vi "Read Data from converted files.vi"(10 "Open Dialog":bool=TRUE, 11 "File Control":path) -> (1 "data":dbl[][](array[numeric]), 3 "dates":string[](array[string]), 5 "File path":path)   [LabVIEW 2018]
uses:
  <vilib>/Utility/file.llb/Read From Spreadsheet File (string).vi
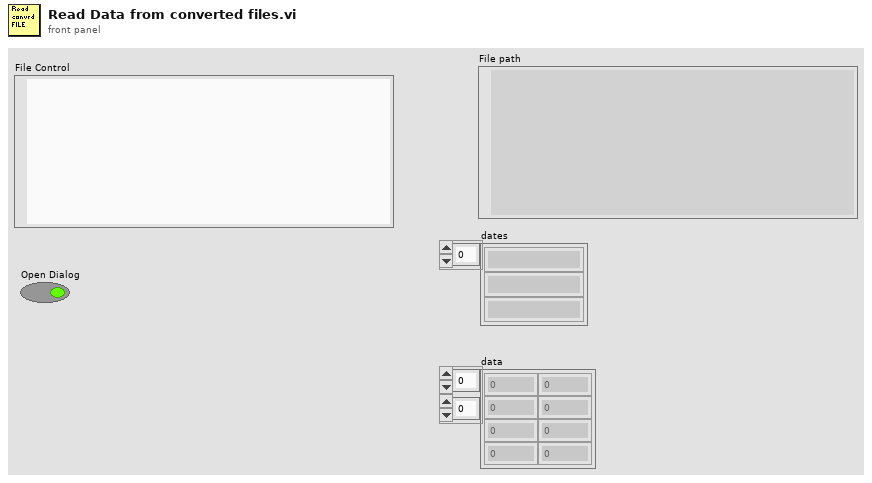
[diagram p1: front panel]
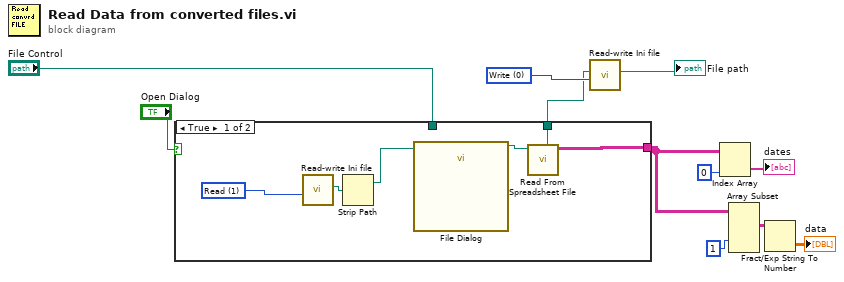
[diagram p0: block diagram]
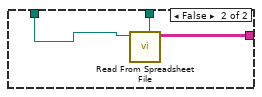
[diagram p2: hidden frame]
diagram:
  w3 = u16 0 items=["Write", "Read"] ("OPERATION")
  n1 = case shown="True" "Open Dialog" {
    tunnel: [w16 w20] -> w8
    tunnel: "File Control" -> [_ w19]
    tunnel: [w15 w18] -> w2
    frame True {
      w14 = u16 1 items=["Write", "Read"] ("OPERATION")
      n2 = call "Read-write Ini file.vi"("OPERATION"=w14) -> ("LAST DATA FILE 2"=w13:path)  [unwired: 10 in]
      n3 = Strip Path(path=w13) -> (stripped path=w12:path)  [unwired: 1 out]
      n4 = call "File Dialog"("start path"=w12) -> ("selected path"=w17:path)  [unwired: 11 in, 3 out]
      n5 = call-poly <vilib>:"Read From Spreadsheet File.vi"("file path (dialog if empty)"=w17) -> ("all rows"=w16:string[][], "new file path (Not A Path if cancelled)"=w15:path)  [unwired: 6 in, 3 out]
    }
    frame False {
      n6 = call-poly <vilib>:"Read From Spreadsheet File.vi"("file path (dialog if empty)"=w19) -> ("all rows"=w20:string[][], "new file path (Not A Path if cancelled)"=w18:path)  [unwired: 6 in, 3 out]
    }
  }
  n7 = call "Read-write Ini file.vi"("OPERATION"=w3, "LAST DATA FILE"=w2) -> ("LAST DATA FILE 2"=→"File path":path)  [unwired: 9 in]
  n8 = Index Array(array=w8, index (col)=0 ("disabled index (col)")) -> (element=→"dates":string[])  [unwired: 1 in]
  n9 = Array Subset(array=w8, index (col)=1 ("length")) -> (w7:string[][])  [unwired: 3 in]
  n10 = Fract/Exp String To Number(string=w7) -> (number=→"data":dbl[][])  [unwired: 3 in, 1 out]
